vi "ex_SignalsToSprdsheetStr.vi"(5 "delimiter (Tab)":string="\t", 6 "Flags":T1={"include col headings?"=TRUE, "x_columns"=0, "col headings always?"=TRUE, "time preference"=0, "hide col headings"=FALSE} {"time preference" items=["Absolute", "Relative"]; "x_columns" items=["None", "One", "Multiple"]}, 8 "error in (no error)":errorcluster, 9 "Decimal Separator":string="%;%g", 10 "comment":string, 11 "Signals":waveform(dbl)[](array[waveform])) -> (0 "error out":errorcluster, 3 "spreadsheet string":string)   [LabVIEW 2020]
uses:
  express input/ExFileReadBlock.llb/ex_ReadFileParams.ctl
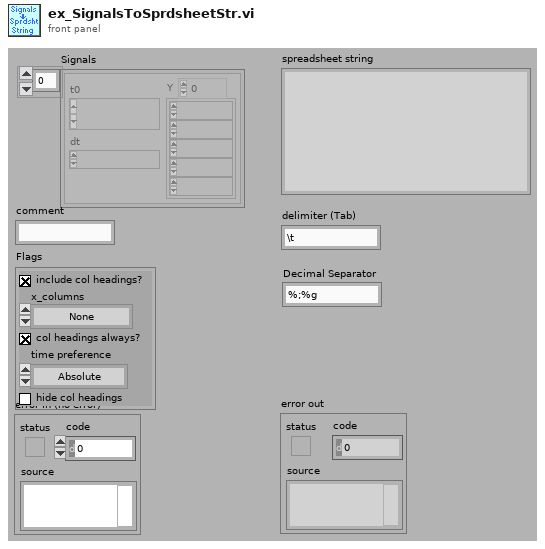
[diagram p1: front panel]
types:
  T1 = typedef "ex_ReadFileParams.ctl" = cluster{"include col headings?":bool, "x_columns":u16, "col headings always?":bool, "time preference":u16, "hide col headings":bool}
  T2 = cluster{"Start Timestamp":timestamp, "Timestamp":timestamp, "Relative Time?":bool, "X Dimension":string, "Signal Name":string, "Y Units":string, "X0":timestamp, "dX":dbl, "nPoints":i32}[]
  T3 = typedef "ex_WaveformAttribsPlus.ctl" = cluster{"Start Timestamp":timestamp, "Timestamp":timestamp, "Relative Time?":bool, "X Dimension":string, "Signal Name":string, "Y Units":string, "X0":timestamp, "dX":dbl, "nPoints":i32}
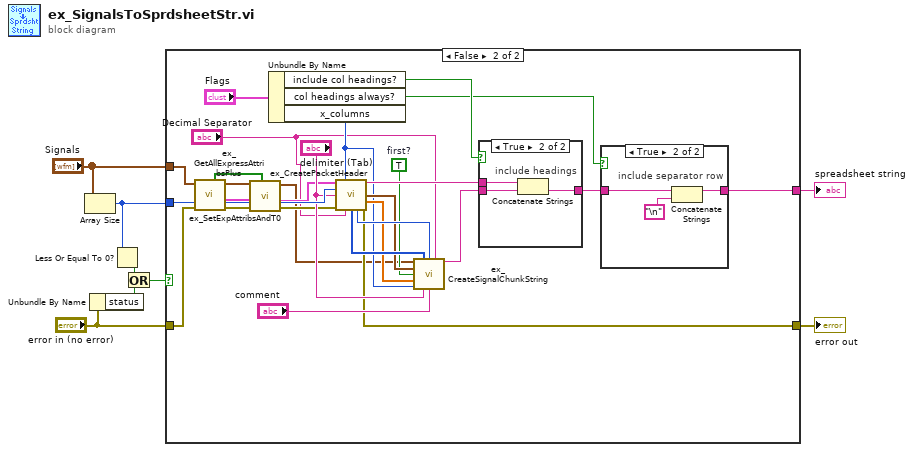
[diagram p0: block diagram]
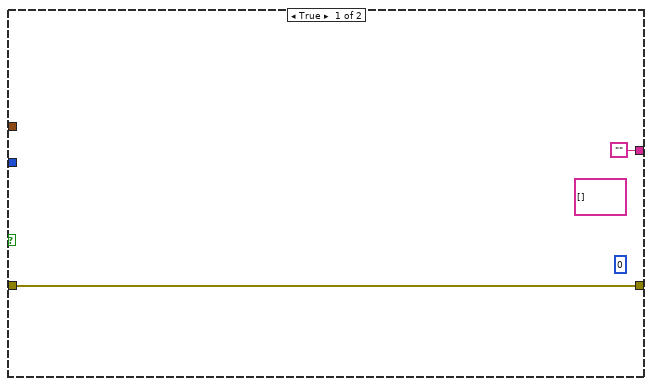
[diagram p2: hidden frame]
diagram:
  n1 = Array Size(array="Signals") -> (size(s)=w6:i32)
  n2 = Unbundle By Name("error in (no error)") -> ("status"=w4:bool)
  n3 = Less Or Equal To 0?(x=w6) -> (x <= 0?=w3:bool)
  n4 = Or(x=w3, y=w4) -> (x .or. y?=w2:bool)
  n5 = case shown="False" w2 {
    tunnel: [w10 w20] -> w8
    tunnel: "error in (no error)" -> [w10 w21]
    tunnel: ["" ("spreadsheet string") w37] -> w7
    tunnel: "Signals" -> [_ w22]
    tunnel: w6 -> [_ w33]
    frame True {
      (unwired) string[][] [] ("string array")
      (unwired) 0
      # "Error or no signals"
    }
    frame False {
      w23 = TRUE  # first?
      n6 = call "ex_GetAllExpressAttribsPlus.vi"("error in"=w21, "Signals in"=w22) -> ("error out"=w19:errorcluster, "All Express Wave Attributes Plus"=w18:T2, "Signals out"=w17:waveform(dbl)[], "Time Attribs Not Found"=w16:bool[])  [unwired: 6 out]
      n7 = call "ex_SetExpAttribsAndT0.vi"("Set? (T if empty)"=w16, "error in (no error)"=w19, "Express Attributes Plus in"=w18, "Signals"=w17) -> ("error out"=w14:errorcluster, "Express Wave Attributes Plus out"=w15:T3[], "Signals With Attributes"=w12:waveform(dbl)[])  [unwired: 2 in, 3 out]
      n8 = Unbundle By Name("Flags") -> ("include col headings?"=w36:bool, "col headings always?"=w34:bool, "x_columns"=w26:u16)
      n9 = call "ex_CreatePacketHeader.vi"("Attributes"=w15, "x_columns"=w26, "nChannels"=w33, "delimiter (Tab)"="delimiter (Tab)", "error in (no error)"=w14, "Decimal Separator"="Decimal Separator") -> ("spreadsheet string"=w32:string, "X0 array"=w28:timestamp[], "dX array"=w27:dbl[], "nPoints array"=w29:i32[], "max nPoints index"=w30:i32, "error out"=w20:errorcluster)  [unwired: 3 in, 1 out]
      n10 = call "ex_CreateSignalChunkString.vi"("Signals"=w12, "nPoints array"=w29, "max nPoints index"=w30, "Decimal Separator"="Decimal Separator", "X0 array"=w28, "first?"=w23, "dX array"=w27, "x_columns"=w26, "delimiter (Tab)"="delimiter (Tab)", "comment"="comment") -> ("spreadsheet string"=w31:string)  [unwired: 1 in, 4 out]
      n11 = case shown="True" w36 {
        tunnel: w32 -> [_ w45]
        tunnel: w31 -> [w42 w44]
        tunnel: [w42 w43] -> w35
        frame False {
          # "omit headings"
        }
        frame True {
          # "include headings"
          n12 = Concatenate Strings(w45, w44) -> (w43:string)
        }
      }
      n13 = case shown="True" w34 {
        tunnel: w35 -> [w38 w41]
        tunnel: [w38 w39] -> w37
        frame False {
        }
        frame True {
          # "include separator row"
          n14 = Concatenate Strings(w41, "\n") -> (w39:string)
        }
      }
    }
  }
  "error out" <- w8
  "spreadsheet string" <- w7
